vi "Make unique panel name.vi"(8 "error in (no error)":errorcluster, 11 "Fiber Auto Collimation panel in":refnum<class "Fiber Auto Collimation panel.lvclass">) -> (0 "error out":errorcluster, 2 "Unique panel name":string, 3 "Fiber Auto Collimation panel out":refnum<class "Fiber Auto Collimation panel.lvclass">)   [LabVIEW 2018, in "Fiber Auto Collimation panel.lvclass"]
doc: "This VI generates a unique name for the panel of the class wired into it.\n\nIf the class wired in supports cloned panels, then the unique name will be based on both the class name and the clone name. If the panel isn't cloneable, then the uniqe name will just be based on the class.\n\nIn both cases, the panel class name (and its clone name) will be made all lowercase so that the names are not case sensitive."
uses:
  Fiber Auto Collimation panel.lvclass
  Fiber Auto Collimation panel.lvclass/Fiber Auto Collimation panel.ctl
  <vilib>/Utility/LVClass/Get LV Class Name.vi
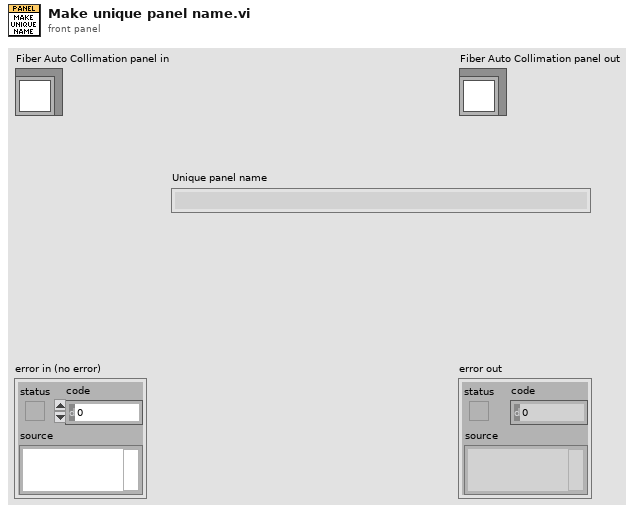
[diagram p1: front panel]
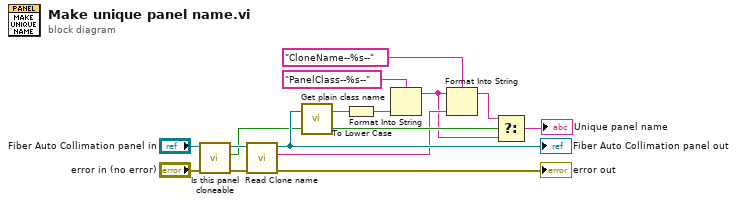
[diagram p0: block diagram]
diagram:
  n1 = call-dynamic "Is this panel cloneable.vi"("error in (no error)"="error in (no error)", "Fiber Auto Collimation panel in"="Fiber Auto Collimation panel in") -> ("error out"=w14:errorcluster, "This class is cloneable"=w9:bool, "Fiber Auto Collimation panel out"=w11:refnum<class "Fiber Auto Collimation panel.lvclass">)  [unwired: 7 in]
  n2 = call "Read Clone name.vi"("error in (no error)"=w14, "Fiber Auto Collimation panel in"=w11) -> ("error out"=→"error out":errorcluster, "Clone name"=w4:string, "Fiber Auto Collimation panel out"=w10:refnum<class "Fiber Auto Collimation panel.lvclass">)  [unwired: 7 in]
  "Fiber Auto Collimation panel out" <- w10
  n3 = call <userlib>:"Get plain class name.vi"("Any class"=w10) -> ("Plain class name"=w7:string)  [unwired: 2 in]
  n4 = To Lower Case(string=w7) -> (all lower case string=w6:string)
  n5 = Format Into String(format string="PanelClass--%s--", w6) -> (resulting string=w1:string)  [unwired: 2 in, 1 out]
  n6 = Format Into String(format string="CloneName--%s--", initial string=w1, w4) -> (resulting string=w2:string)  [unwired: 1 in, 1 out]
  n7 = Select(t=w2, s=w9, f=w1) -> (s? t:f=→"Unique panel name":string)
